vi "PUT Sample Rate.vi"(0 "Calibration Sample Rate":dbl) -> ()   [LabVIEW 2013]
uses:
  Action.ctl
  Calibration Input FGV Selector.ctl
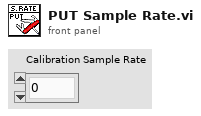
[diagram p1: front panel]
types:
  T1 = typedef "Calibration Input FGV Selector.ctl" = enum16{"Samples/Sweep", "Num Sweeps", "Sample Rate"}
  T2 = typedef "Action.ctl" = enum16{"GET", "PUT", "DELETE"}
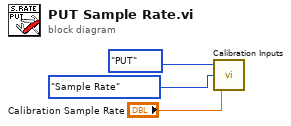
[diagram p0: block diagram]
diagram:
  n1 = call "Calibration Inputs.vi"("Input"="Calibration Sample Rate", "Calibration Input FGV Selector"=Calibration_Input_FGV_Selector."Sample Rate", "Verb"=Action."PUT") -> ()  [unwired: 1 out]
